vi "Run.vi"(8 "error in (no error)":errorcluster, 11 "VIEW in":refnum<class "VIEW.lvclass">) -> (0 "error out":errorcluster, 3 "VIEW out":refnum<class "VIEW.lvclass">)   [LabVIEW 2013, in "VIEW.lvclass"]
uses:
  VIEW.lvclass
  VIEW.lvclass/VIEW.ctl
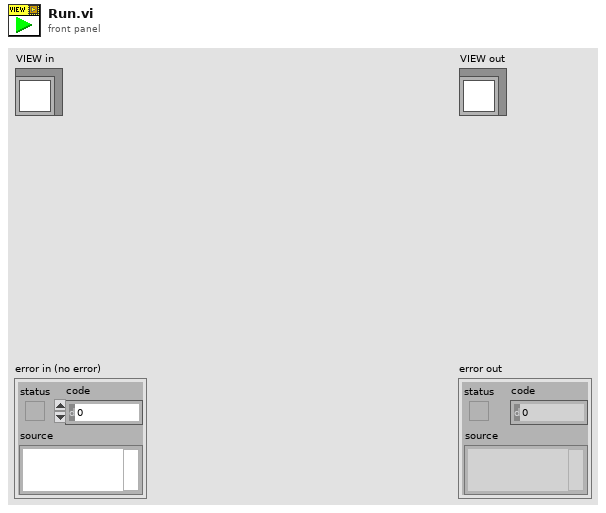
[diagram p1: front panel]
types:
  T1 = enum32{"Invalid", "Standard", "Closed", "Hidden", "Minimized", "Maximized"}
  T2 = enum32{"Bad", "Idle", "Run top level", "Running"}
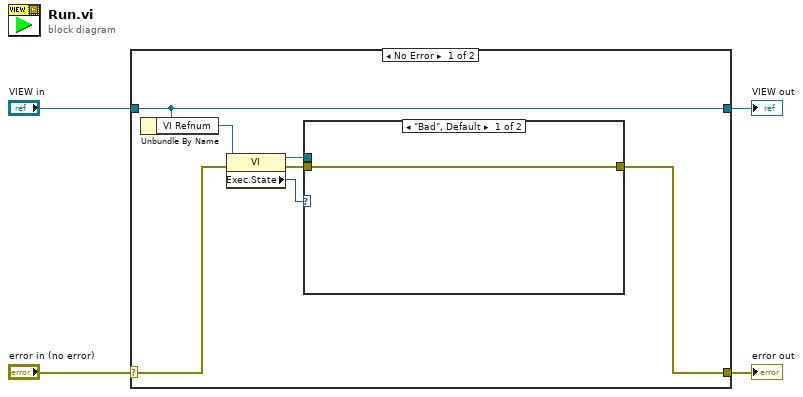
[diagram p0: block diagram]
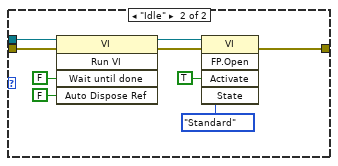
[diagram p2: hidden frame]
diagram:
  n1 = case shown="No Error" "error in (no error)" {
    selector: "error in (no error)" -> [w5 w23]
    tunnel: [w10 w23] -> w3
    tunnel: [w11 w22] -> w1
    tunnel: "VIEW in" -> [w11 w22]
    frame No Error {
      n2 = Unbundle By Name(w11) -> ("VI Refnum"=w8:refnum<vi>)
      n3 = property class="VI"(reference=w8, error in=w5) -> (reference out=w7:refnum<vi>, error out=w6:errorcluster, "Exec.State"=w9:T2)
      n4 = case shown="\"Bad\", Default" w9 {
        tunnel: w7 -> [_ w21]
        tunnel: w6 -> [w12 w18]
        tunnel: [w12 w13] -> w10
        frame "Bad", Default {
        }
        frame "Idle" {
          n5 = invoke class="VI" method="Run VI"(reference=w21, error in=w18, "Wait until done"=FALSE ("Wait Until Done"), "Auto Dispose Ref"=FALSE ("Auto Dispose Reference")) -> (reference out=w16:refnum<vi>, error out=w17:errorcluster)  [unwired: 1 in, 3 out]
          n6 = invoke class="VI" method="FP.Open"(reference=w16, error in=w17, "Activate"=TRUE ("Activate?"), "State"=T1."Standard") -> (error out=w13:errorcluster)  [unwired: 1 in, 4 out]
        }
      }
    }
    frame Error {
    }
  }
  "error out" <- w3
  "VIEW out" <- w1
